vi "Append Node to XML.vi"(4 "Data":string, 6 "Tag Name":string, 9 "SuperElement In":refnum<k20>, 10 "error in":errorcluster, 11 "DOM document in":refnum<k20>) -> (1 "SuperElement Out":refnum<k20>, 2 "error out":errorcluster, 3 "DOM document out":refnum<k20>)   [LabVIEW 2013]
uses:
  <resource>/objmgr/DOMUserDefRef.rc
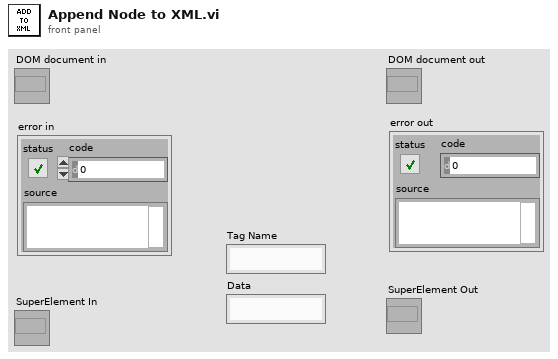
[diagram p1: front panel]
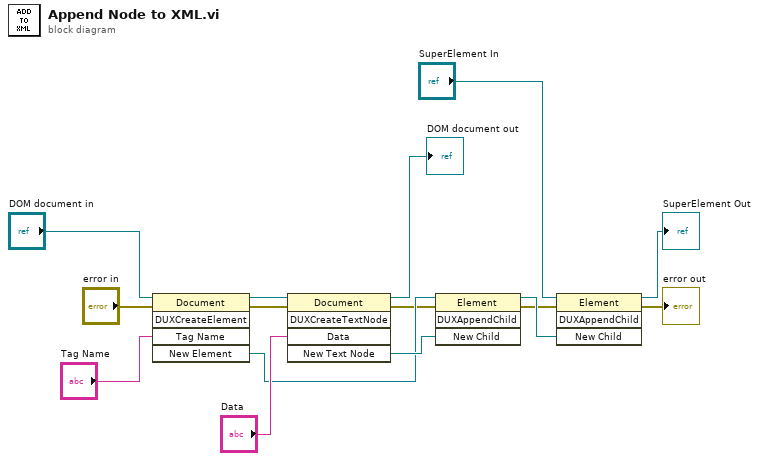
[diagram p0: block diagram]
diagram:
  n1 = invoke class="Document" method="DUXCreateElement"(reference="DOM document in", error in="error in", "Tag Name"="Tag Name") -> (reference out=w9:refnum<k20>, error out=w4:errorcluster, "New Element"=w8:refnum<k20>)  [unwired: 2 in, 2 out]
  n2 = invoke class="Document" method="DUXCreateTextNode"(reference=w9, error in=w4, "Data"="Data") -> (reference out=→"DOM document out":refnum<k20>, error out=w3:errorcluster, "New Text Node"=w11:refnum<k20>)  [unwired: 2 in, 2 out]
  n3 = invoke class="Element" method="DUXAppendChild"(reference=w8, error in=w3, "New Child"=w11) -> (reference out=w6:refnum<k20>, error out=w2:errorcluster)  [unwired: 1 in, 2 out]
  n4 = invoke class="Element" method="DUXAppendChild"(reference="SuperElement In", error in=w2, "New Child"=w6) -> (reference out=→"SuperElement Out":refnum<k20>, error out=→"error out":errorcluster)  [unwired: 1 in, 2 out]
